vi "Waveform ppsu.vi"(11 "Array in":dbl[](array[numeric])) -> (3 "Array out":waveform(dbl)[](array[waveform]))   [LabVIEW 2022 SP3]
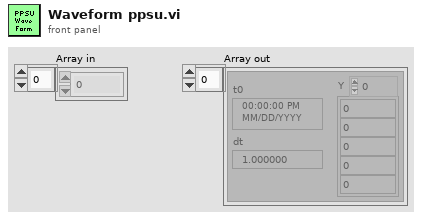
[diagram p1: front panel]
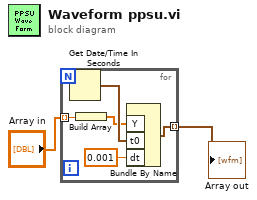
[diagram p0: block diagram]
diagram:
  n1 = for {
    tunnel: [w7] -> w1 mode=indexing
    tunnel: "Array in" -> [w4] mode=indexing
    n2 = Get Date/Time In Seconds() -> (seconds since 1Jan1904=w6:timestamp)
    n3 = Build Array(w4) -> (w3:dbl[])
    n4 = Bundle By Name("Y"=w3, "t0"=w6, "dt"=0.001) -> (w7:waveform(dbl))  [unwired: 1 in]
  }
  "Array out" <- w1
